vi "Autonomous Independent.vi"() -> ()   [LabVIEW 2013]
doc: "This VI is called when autonomous begins, and will automatically be terminated when autonomous ends. You can carry out timed or sensor driven robot movement independently without needing to return to the caller."
uses:
  Robot Global Data.vi
  <vilib>/Rock Robotics/WPI/Joystick/WPI_JoystickGetSetRefNum.vi
  <vilib>/Rock Robotics/WPI/RobotDrive/WPI_RobotDriveArcadeDrive_Standard(NoSaturation).vi
panel:
  out "Accel Sensor":dbl
  out "Gyro Sensor":dbl
  out "Sonic Sensor":dbl
  out "Current Movement, for debugging":T1 {"Y Joystick Value" scale=1.0..-1.0; "X Joystick Value" scale=-1.0..1.0}
  in  "Array of robot movements":T2(array[cluster]) {"Y Joystick Value" scale=1.0..-1.0; "X Joystick Value" scale=-1.0..1.0}
  # "Be sure to right-click and choose Data Operations>>Make Current Value default if you want to save the array values with the VI"
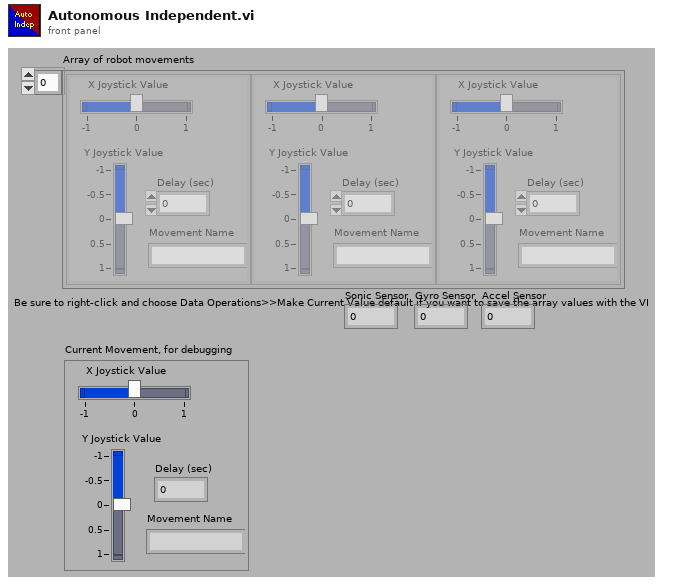
[diagram p1: front panel]
types:
  T1 = cluster{"X Joystick Value":dbl, "Y Joystick Value":dbl, "Delay (sec)":dbl, "Movement Name":string}
  T2 = cluster{"X Joystick Value":dbl, "Y Joystick Value":dbl, "Delay (sec)":dbl, "Movement Name":string}[]
  T3 = enum16{"START", "TWO", "THREE", "FOUR", "FIVE", "SIX", "END"}
  T4 = typedef "WPI_JoystickDevRef.ctl" = cluster{"Device":T5}
  T5 = typedef "WPI_JoystickDeviceEnum.ctl" = enum16{"USB 1", "USB 2", "USB 3", "USB 4", "Kinect 1", "Kinect 2"}
  T6 = cluster{"axis 1 (x)":dbl, "axis 2 (y)":dbl, "axis 3 (throttle)":dbl, "axis 4":dbl, "axis 5":dbl, "axis 6":dbl}
  T7 = typedef "WPI_RobotDriveDevRef.ctl" = cluster{"DevStatus":errorcluster, "Motors[]":T8[], "Square Inputs":bool, "Max Output":dbl, "Isochronous":bool}
  T8 = typedef "WPI_MotorControlDeviceRef.ctl" = cluster{"DeviceStatus":errorcluster, "Type":enum16{"PWM", "CAN"}, "PWM":cluster{"Digital Module":T9, "PWM Channel":T10, "DeadBand":T11}, "CAN":cluster{"Device Number":u8, "Control Mode":T12, "Semaphore":T13, "Max Vout":dbl}, "Invert":bool, "TransformRef":T14, "InvTransformRef":T14}
  T9 = typedef "FPGA_TypedefDigitalModule.ctl" = enum16{"Digital Module 1", "Digital Module 2"}
  T10 = typedef "FPGA_DIOPWMChannel.ctl" = enum8{"PWM 1", "PWM 2", "PWM 3", "PWM 4", "PWM 5", "PWM 6", "PWM 7", "PWM 8", "PWM 9", "PWM 10", "Invalid"}
  T11 = typedef "WPI_PWMDeadband.ctl" = cluster{"Name":string, "maxPositivePwm":i32, "minPositivePwm":i32, "centerPwm":i32, "maxNegativePwm":i32, "minNegativePwm":i32, "angularRange":u16}
  T12 = typedef "WPI_CANJaguar_ControlMode.ctl" = enum8{"Percent VBus", "Current", "Speed", "Position", "Voltage"}
  T13 = typedef "Semaphore RefNum" = refnum<k1>
  T14 = typedef "WPI_PWMTransform_ConPane.ctl" = refnum<vi>
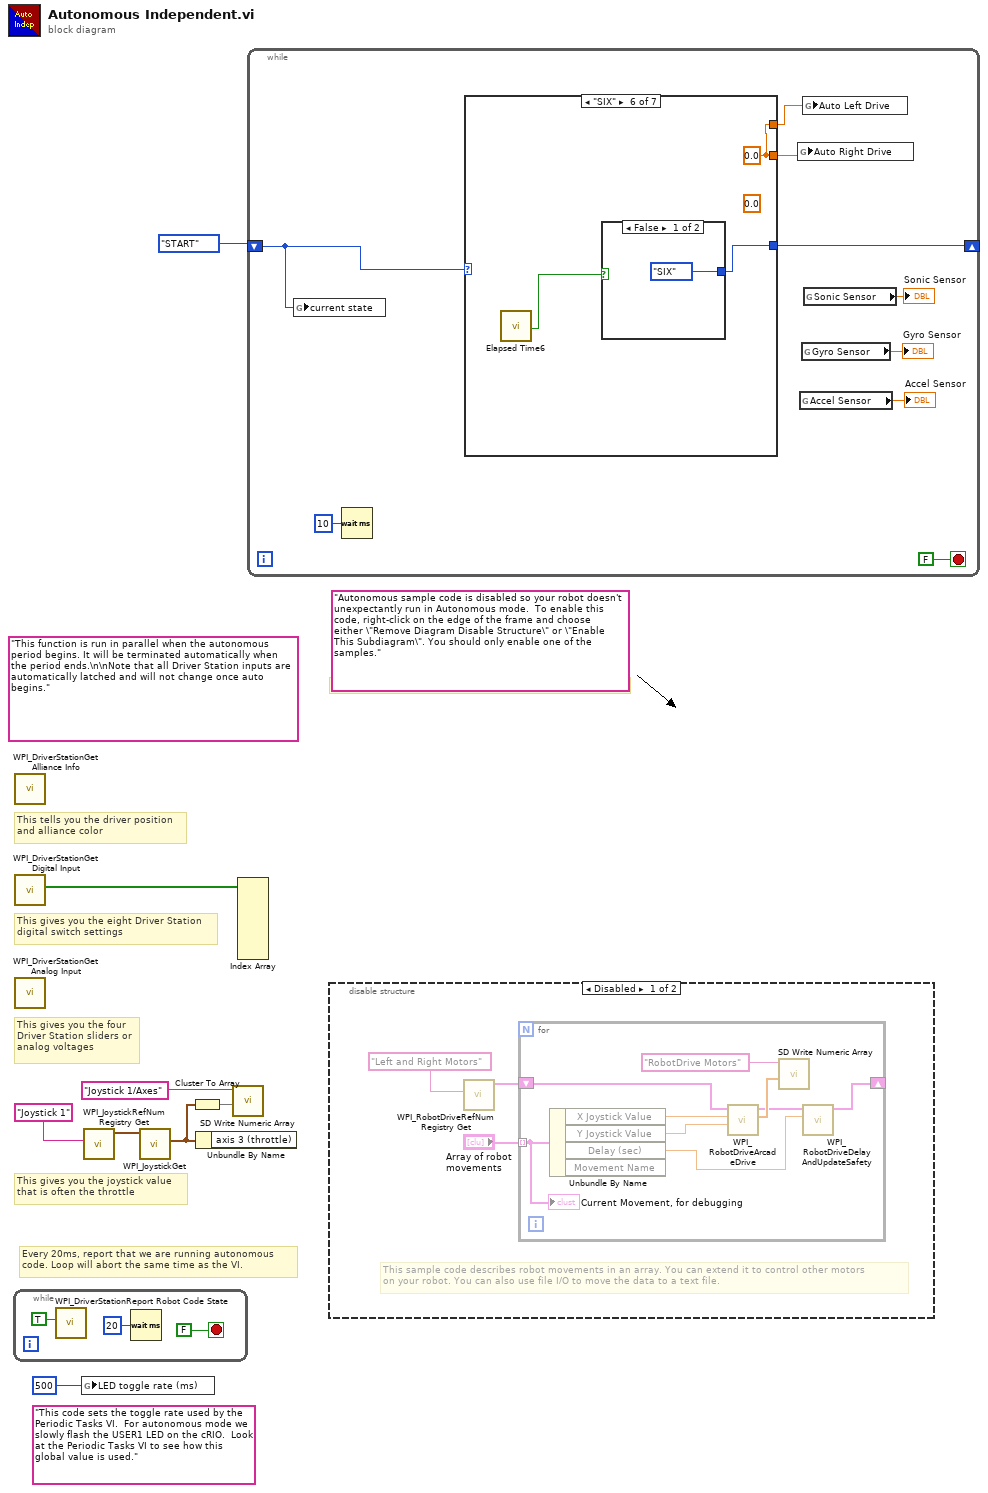
[diagram p0: block diagram]
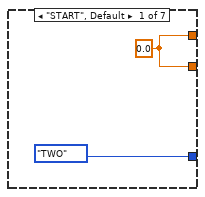
[diagram p2: hidden frame]
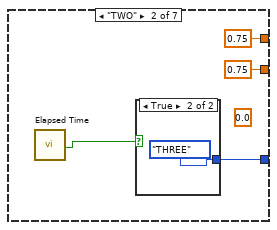
[diagram p3: hidden frame]
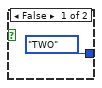
[diagram p4: hidden frame]
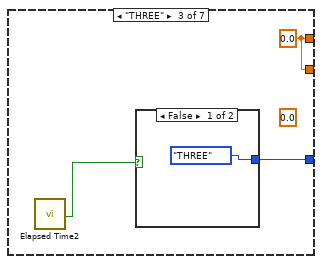
[diagram p5: hidden frame]
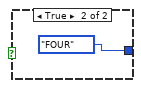
[diagram p6: hidden frame]
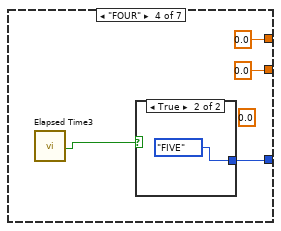
[diagram p7: hidden frame]
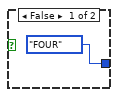
[diagram p8: hidden frame]
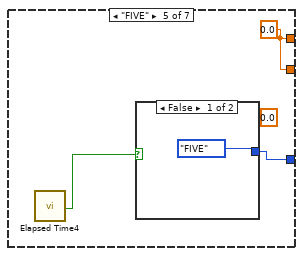
[diagram p9: hidden frame]
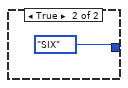
[diagram p10: hidden frame]
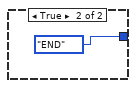
[diagram p11: hidden frame]
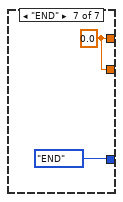
[diagram p12: hidden frame]
diagram:
  (unwired) "This code sets the toggle rate used by the Periodic Tasks VI.  For autonomous mode we slowly flash the USER1 LED on the cRIO.  Look at the Periodic Tasks VI to see how this global value is used."
  (unwired) "Autonomous sample code is disabled so your robot doesn't unexpectantly run in Autonomous mode.  To enable this code, right-click on the edge of the frame and choose either \"Remove Diagram Disable Structure\" or \"Enable This Subdiagram\". You should only enable one of the samples."
  (unwired) "This function is run in parallel when the autonomous period begins. It will be terminated automatically when the period ends.\n\nNote that all Driver Station inputs are automatically latched and will not change once auto begins."
  # "Every 20ms, report that we are running autonomous\ncode. Loop will abort the same time as the VI."
  # "This gives you the joystick value\nthat is often the throttle"
  # "Use time and/or sensors to control how the robot drives."
  # "This tells you the driver position\nand alliance color"
  # "This gives you the eight Driver Station\ndigital switch settings"
  # "This gives you the four\nDriver Station sliders or\nanalog voltages"
  n1 = while {
    stop <- FALSE stop-if-true
    n2 = call <vilib>:"WPI_DriverStationReport Robot Code State.vi"("Autonomous"=TRUE) -> ()  [unwired: 10 in, 1 out]
    n3 = Wait (ms)(milliseconds to wait=u32 20) -> ()  [unwired: 1 out]
  }
  n4 = call <vilib>:"WPI_DriverStationGet Alliance Info.vi"() -> ()  [unwired: 12 out]
  n5 = call <vilib>:"WPI_DriverStationGet Digital Input.vi"() -> ("Driver Station Digital Input (1-8)"=w8:bool[])  [unwired: 11 out]
  n6 = call <vilib>:"WPI_DriverStationGet Analog Input.vi"() -> ()  [unwired: 12 out]
  n7 = global write "Robot Global Data.vi" "LED toggle rate (ms)"(u32 500 ("LED ms toggle rate")) -> ()
  n8 = call <vilib>:"WPI_JoystickRefNum Registry Get.vi"("refnum name"="Joystick 1") -> ("JoystickDevRef"=w6:T4)  [unwired: 1 in, 9 out]
  n9 = call <vilib>:"WPI_JoystickGet.vi"("JoystickDevRef"=w6) -> ("Axes"=w3:T6)  [unwired: 1 in, 5 out]
  n10 = Cluster To Array(cluster=w3) -> (array=w4:dbl[])
  n11 = Unbundle By Name(w3) -> ()  [unwired: 1 out]
  n12 = call <vilib>:"SD Write Numeric Array.vi"("Numeric Array"=w4, "Name"="Joystick 1/Axes") -> ()  [unwired: 8 in, 2 out]
  n13 = Index Array(array=w8) -> ()  [unwired: 8 in, 8 out]
  n14 = while {
    shift-right: [w19] -> _
    shift-left: T3."START" -> [w18]
    stop <- FALSE stop-if-true
    n15 = global write "Robot Global Data.vi" "current state"(w18) -> ()
    n16 = Wait (ms)(milliseconds to wait=u32 10) -> ()  [unwired: 1 out]
    n17 = case shown="\"SIX\"" w18 {
      tunnel: [w22 0.75 ("Auto Right Drive") w29 0.0 ("Auto Right Drive") w40 w47 w50] -> w16
      tunnel: [w22 0.75 ("Auto Right Drive") w29 0.0 ("Auto Right Drive") w40 w47 w50] -> w15
      tunnel: [T3."TWO" w24 w30 w36 w41 w45 T3."END"] -> w19
      frame "START", Default {
        w22 = 0.0 ("Auto Right Drive")
      }
      frame "TWO" {
        (unwired) 0.0 ("Arm Drive")
        n18 = call "Elapsed Time"() -> ("Time has Elapsed"=w23:bool)  [unwired: 12 in, 7 out]
        n19 = case shown="True" w23 {
          tunnel: [T3."TWO" T3."THREE"] -> w24
          frame False {
          }
          frame True {
          }
        }
      }
      frame "THREE" {
        (unwired) 0.0 ("Arm Drive")
        w29 = 0.0 ("Auto Right Drive")
        n20 = call "Elapsed Time2"() -> ("Time has Elapsed"=w31:bool)  [unwired: 12 in, 7 out]
        n21 = case shown="False" w31 {
          tunnel: [T3."THREE" T3."FOUR"] -> w30
          frame False {
          }
          frame True {
          }
        }
      }
      frame "FOUR" {
        (unwired) 0.0 ("Arm Drive")
        n22 = call "Elapsed Time3"() -> ("Time has Elapsed"=w37:bool)  [unwired: 12 in, 7 out]
        n23 = case shown="True" w37 {
          tunnel: [T3."FOUR" T3."FIVE"] -> w36
          frame False {
          }
          frame True {
          }
        }
      }
      frame "FIVE" {
        (unwired) 0.0 ("Arm Drive")
        w40 = 0.0 ("Auto Right Drive")
        n24 = call "Elapsed Time4"() -> ("Time has Elapsed"=w42:bool)  [unwired: 12 in, 7 out]
        n25 = case shown="False" w42 {
          tunnel: [T3."FIVE" T3."SIX"] -> w41
          frame False {
          }
          frame True {
          }
        }
      }
      frame "SIX" {
        (unwired) 0.0 ("Arm Drive")
        w47 = 0.0 ("Auto Right Drive")
        n26 = call "Elapsed Time6"() -> ("Time has Elapsed"=w46:bool)  [unwired: 12 in, 7 out]
        n27 = case shown="False" w46 {
          tunnel: [T3."SIX" T3."END"] -> w45
          frame False {
          }
          frame True {
          }
        }
      }
      frame "END" {
        w50 = 0.0 ("Auto Right Drive")
      }
    }
    n28 = global write "Robot Global Data.vi" "Auto Right Drive"(w15) -> ()
    n29 = global read "Robot Global Data.vi" "Accel Sensor"() -> (→"Accel Sensor":dbl)
    n30 = global read "Robot Global Data.vi" "Gyro Sensor"() -> (→"Gyro Sensor":dbl)
    n31 = global write "Robot Global Data.vi" "Auto Left Drive"(w16) -> ()
    n32 = global read "Robot Global Data.vi" "Sonic Sensor"() -> (→"Sonic Sensor":dbl)
  }
  n33 = disable-structure shown="Disabled" {
    frame Disabled {
      # "This sample code describes robot movements in an array. You can extend it to control other motors\non your robot. You can also use file I/O to move the data to a text file."
      n34 = call <vilib>:"WPI_RobotDriveRefNum Registry Get.vi"("refnum name"="Left and Right Motors") -> ("RobotDriveDevRef"=w53:T7)  [unwired: 1 in, 9 out]
      n35 = for {
        shift-right: [w59] -> _
        shift-left: w53 -> [w60]
        tunnel: "Array of robot movements" -> [w55] mode=indexing
        n36 = Unbundle By Name(w55) -> ("X Joystick Value"=w58:dbl, "Y Joystick Value"=w57:dbl, "Delay (sec)"=w56:dbl)  [unwired: 1 out]
        n37 = call-poly <vilib>:"WPI_RobotDriveArcadeDrive.vi"("Y axis value"=w57, "X axis value"=w58, "RobotDriveDevRef"=w60) -> ("Motor Values"=w62:dbl[], "RobotDriveDevRef"=w61:T7)  [unwired: 1 in, 6 out]
        n38 = call <vilib>:"SD Write Numeric Array.vi"("Numeric Array"=w62, "Name"="RobotDrive Motors") -> ()  [unwired: 8 in, 2 out]
        n39 = call <vilib>:"WPI_RobotDriveDelayAndUpdateSafety.vi"("Delay (s)"=w56, "RobotDriveDevRef"=w61) -> ("RobotDriveDevRef 2"=w59:T7)  [unwired: 8 in, 1 out]
        "Current Movement, for debugging" <- w55
      }
    }
    frame Enabled {
    }
  }
